vi "cmdElements2Text.vi"(1 "CodeElements":T3={"address"="010000000000", "controlCode"="11", "dataLength"=4.0, "dataSection"="12345678", "checkCode"="7F"}) -> (0 "CommandText":T1)   [LabVIEW 2010]
uses:
  OutputDataFormat.ctl
  <vilib>/xml/Load XML File.vi
  <vilib>/xml/NI_XML.lvlib
  Program Files/National Instruments/LabVIEW 2010/resource/objmgr/DOMUserDefRef.rc
panel:
  out "TextElements":T2
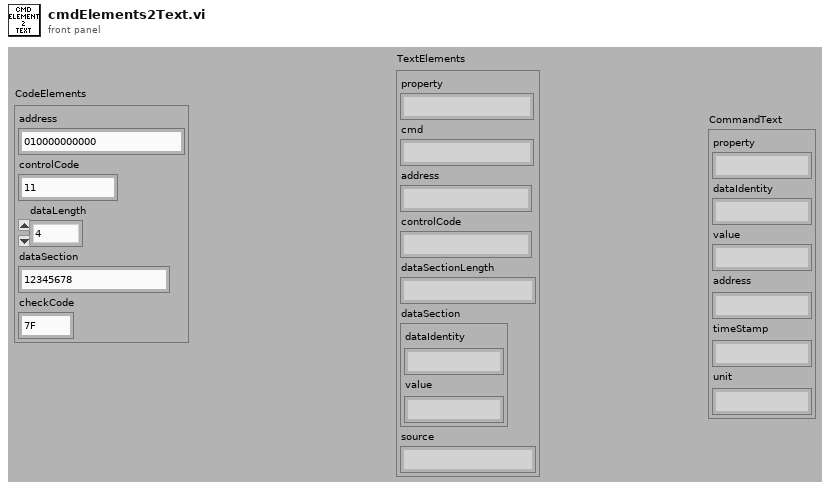
[diagram p1: front panel]
types:
  T1 = typedef "OutputDataFormat.ctl" = cluster{"property":string, "dataIdentity":string, "value":string, "address":string, "timeStamp":string, "unit":string}
  T2 = cluster{"property":string, "cmd":string, "address":string, "controlCode":string, "dataSectionLength":string, "dataSection":cluster{"dataIdentity":string, "value":string}, "source":string}
  T3 = cluster{"address":string, "controlCode":string, "dataLength":dbl, "dataSection":string, "checkCode":string}
  T4 = cluster{"property":string, "cmd":string, "address":string, "controlCode":string, "dataSectionLength":string, "dataSection":string, "source":string}
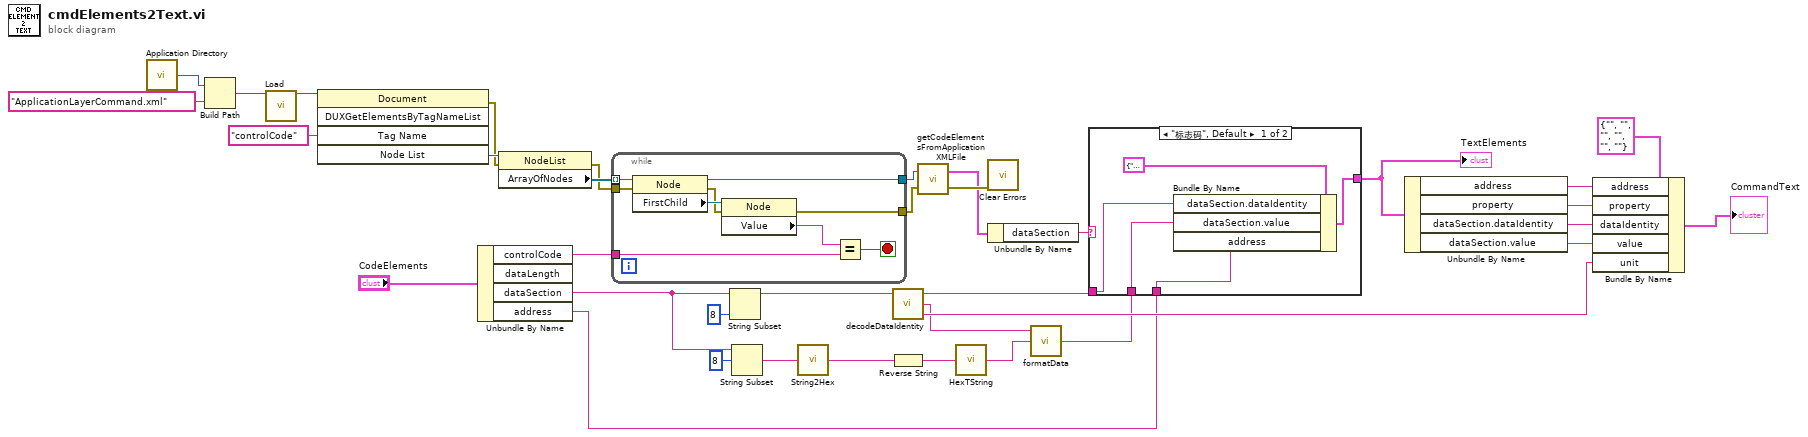
[diagram p0: block diagram]
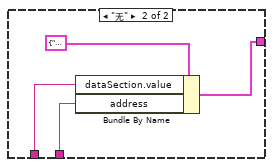
[diagram p2: hidden frame]
diagram:
  n1 = call <vilib>:"Application Directory.vi"() -> ("Application Directory"=w9:path)
  n2 = Build Path(base path=w9, name or relative path="ApplicationLayerCommand.xml") -> (appended path=w7:path)
  n3 = call-poly <vilib>:"Load.vi"("path to XML document"=w7) -> ("DOM document out"=w33:refnum<k20>)  [unwired: 12 in, 2 out]
  n4 = invoke class="Document" method="DUXGetElementsByTagNameList"(reference=w33, "Tag Name"="controlCode") -> (error out=w6:errorcluster, "Node List"=w31:refnum<k20>)  [unwired: 3 in, 3 out]
  n5 = Unbundle By Name("CodeElements") -> ("controlCode"=w30:string, "dataSection"=w19:string, "address"=w25:string)  [unwired: 1 out]
  n6 = property class="NodeList"(reference=w31, error in=w6) -> (error out=w5:errorcluster, "ArrayOfNodes"=w29:refnum<k20>[])  [unwired: 1 out]
  n7 = while {
    tunnel: w30 -> [w44]
    tunnel: w29 -> [w45] mode=indexing
    tunnel: [w41] -> w28
    tunnel: w5 -> [w39]
    tunnel: [w37] -> w4
    stop <- w42 stop-if-true
    n8 = property class="Node"(reference=w45, error in=w39) -> (reference out=w41:refnum<k20>, error out=w38:errorcluster, "FirstChild"=w40:refnum<k20>)
    n9 = property class="Node"(reference=w40, error in=w38) -> (error out=w37:errorcluster, "Value"=w43:string)  [unwired: 1 out]
    n10 = Equal?(x=w43, y=w44) -> (x = y?=w42:bool)
  }
  n11 = String Subset(string=w19, length (rest)=8 ("offset (0)")) -> (substring=w23:string)  [unwired: 1 in]
  n12 = String Subset(string=w19, offset (0)=8) -> (substring=w12:string)  [unwired: 1 in]
  n13 = call "String2Hex.vi"("value"=w12) -> ("String"=w11:string)
  n14 = call "decodeDataIdentity.vi"("dataIdentityCode"=w23) -> ("unit"=w36:string, "dataFormat"=w3:string, "dataIdentityText"=w24:string)  [unwired: 2 in]
  n15 = Reverse String(1:w11) -> (0:w10:string)
  n16 = call "getCodeElementsFromApplicationXMLFile.vi"("error in (no error)"=w4, "Node"=w28) -> ("error out"=w35:errorcluster, "TextElements"=w27:T4)
  n17 = call "HexTString.vi"("input Hex"=w10) -> ("output string"=w2:string)
  n18 = call <vilib>:"Clear Errors.vi"("error in (no error)"=w35) -> ()  [unwired: 6 in, 1 out]
  n19 = Unbundle By Name(w27) -> ("dataSection"=w26:string)
  n20 = call "formatData.vi"("originalData"=w2, "dataFormat"=w3) -> ("formatedData"=w1:string)  [unwired: 2 in, 1 out]
  n21 = case shown="\"标志码\", Default" w26 {
    tunnel: w24 -> [w47 _]
    tunnel: [w50 w53] -> w22
    tunnel: w25 -> [w49 w54]
    tunnel: w1 -> [w46 w51]
    frame "标志码", Default {
      n22 = Bundle By Name(cluster=T2 {"property"="读数据", "cmd"="主站请求帧", "address"="AAAAAAAAAAAA", "controlCode"="11", "dataSectionLength"="04", "dataSection"={"dataIdentity"="", "value"=""}, "source"="主站"} ("TextElements"), "dataSection.dataIdentity"=w47, "dataSection.value"=w46, "address"=w49) -> (w50:T2)
    }
    frame "无" {
      n23 = Bundle By Name(cluster=T2 {"property"="读数据", "cmd"="主站请求帧", "address"="AAAAAAAAAAAA", "controlCode"="11", "dataSectionLength"="04", "dataSection"={"dataIdentity"="", "value"=""}, "source"="主站"} ("TextElements"), "dataSection.value"=w51, "address"=w54) -> (w53:T2)
    }
  }
  "TextElements" <- w22
  n24 = Unbundle By Name(w22) -> ("address"=w13:string, "property"=w18:string, "dataSection.dataIdentity"=w17:string, "dataSection.value"=w16:string)
  n25 = Bundle By Name(cluster=T1 {"property"="", "dataIdentity"="", "value"="", "address"="", "timeStamp"="", "unit"=""} ("CommandText"), "address"=w13, "property"=w18, "dataIdentity"=w17, "value"=w16, "unit"=w36) -> (→"CommandText":T1)
